vi "GetAllTypes.vi"(11 "variables":cluster{"Name":string, "Variant Data":variant}[](array[cluster])) -> (3 "types":cluster{"Name":string, "Type":string}[](array[cluster]))   [LabVIEW 2015]
uses:
  <vilib>/Utility/Data Type/NI_Data Type.lvlib
panel:
  # "GetTypes"
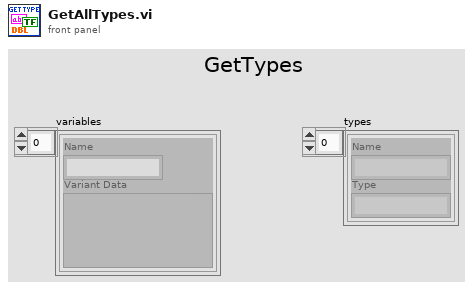
[diagram p1: front panel]
types:
  T1 = typedef "NI_Data Type.lvlib/Data Type.ctl" = enum8{"Invalid Type", "Void", "I8", "I16", "I32", "I64", "U8", "U16", "U32", "U64", "Single Float", "Double Float", "Extended Float", "Single Complex", "Double Complex", "Extended Complex", "Enum U8", "Enum U16", "Enum U32", "Enum U64", "Single Float With Unit", "Double Float With Unit", "Extended Float With Unit", "Single Complex with Unit", "Double Complex with Unit", "Extended Complex with Unit", "Boolean", "String", "Path", "Picture", "Tag", "Array", "Cluster", "Variant", "LV Variant", "Waveform", "Timestamp", "Digital Waveform", "Digital Data", "ExpressData", "Refnum", "External Data", "VI", "Poly VI", "LabVIEW Class Instance", "Fixed Point"}
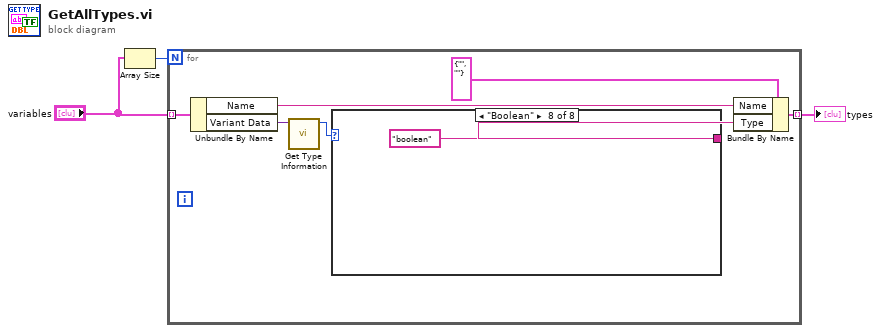
[diagram p0: block diagram]
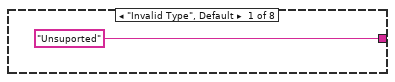
[diagram p2: hidden frame]
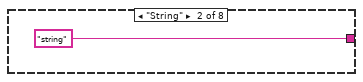
[diagram p3: hidden frame]
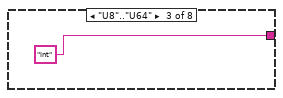
[diagram p4: hidden frame]
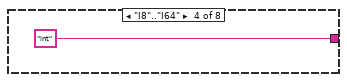
[diagram p5: hidden frame]
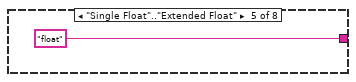
[diagram p6: hidden frame]
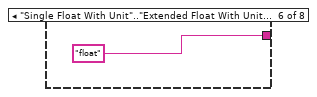
[diagram p7: hidden frame]
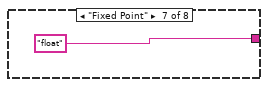
[diagram p8: hidden frame]
diagram:
  n1 = Array Size(array="variables") -> (size(s)=w1:i32)
  n2 = for {
    N: w1 -> [_]
    tunnel: "variables" -> [w10] mode=indexing
    tunnel: [w4] -> w3 mode=indexing
    n3 = Unbundle By Name(w10) -> ("Name"=w7:string, "Variant Data"=w9:variant)
    n4 = call <vilib>:"Get Type Information.vi"("Variant"=w9) -> ("Type"=w8:T1)  [unwired: 6 in, 4 out]
    n5 = case shown="\"Boolean\"" w8 {
      tunnel: ["Unsuported" "string" "int" "int" "float" "float" "float" "boolean"] -> w6
      frame "Invalid Type", Default {
      }
      frame "String" {
      }
      frame "U8".."U64" {
      }
      frame "I8".."I64" {
      }
      frame "Single Float".."Extended Float" {
      }
      frame "Single Float With Unit".."Extended Float With Unit" {
      }
      frame "Fixed Point" {
      }
      frame "Boolean" {
      }
    }
    n6 = Bundle By Name(cluster=cluster{"Name":string, "Type":string} {"Name"="", "Type"=""} ("element"), "Name"=w7, "Type"=w6) -> (w4:cluster{"Name":string, "Type":string})
  }
  "types" <- w3
